vi "4Pi Astigmatism Alignment.vi"(7 "Calling VI Ref":refnum<vi>) -> ()   [LabVIEW 2016]
uses:
  Hardware Configuration/Hardware Configuration Controls/Device Type.ctl
  Hardware Configuration/Hardware Configuration Controls/Device Function.ctl
  <vilib>/Utility/miscctls.llb/LVPointTypeDef.ctl
  4Pi Astigmatism Alignment Type Defs/4Pi AA Actions.ctl
  4Pi Astigmatism Alignment Type Defs/4Pi AA Notifier Type.ctl
  Device Library/Stages/Stages Controls/Stage Actions.ctl
  <vilib>/vision/Image Controls.llb/IMAQ Image.ctl
  Device Library/Cameras/Hamamatsu/Orca Flash/Orca Flash Controls/Orca Flash Actions.ctl
  <vilib>/Analysis/NI_AALPro.lvlib
  <vilib>/Analysis/polynomials.llb/Polynomial Plot (Range).vi
  Device Library/Shutters/Shutter Controls/Shutter Actions.ctl
panel:
  in  "Scan and Align":bool
  in  "Scan Lower Obj":bool
  in  "Frame Accums.":u16=1
  in  "No. of Steps":u16=10
  in  "Step Size (µm)":dbl=0.05
  out "ROI Fit":dbl[][](graph)
  out "Image ROI":u16[][](graph)
  in  "Image Selection":i32(ring) items=["Quad 01", "Quad 02", "Quad 03", "Quad 04"]
  in  "Scan Upper Obj":bool
  in  "Quit":bool
  out "Scan Data":cluster{dbl[], dbl[]}[](graph)
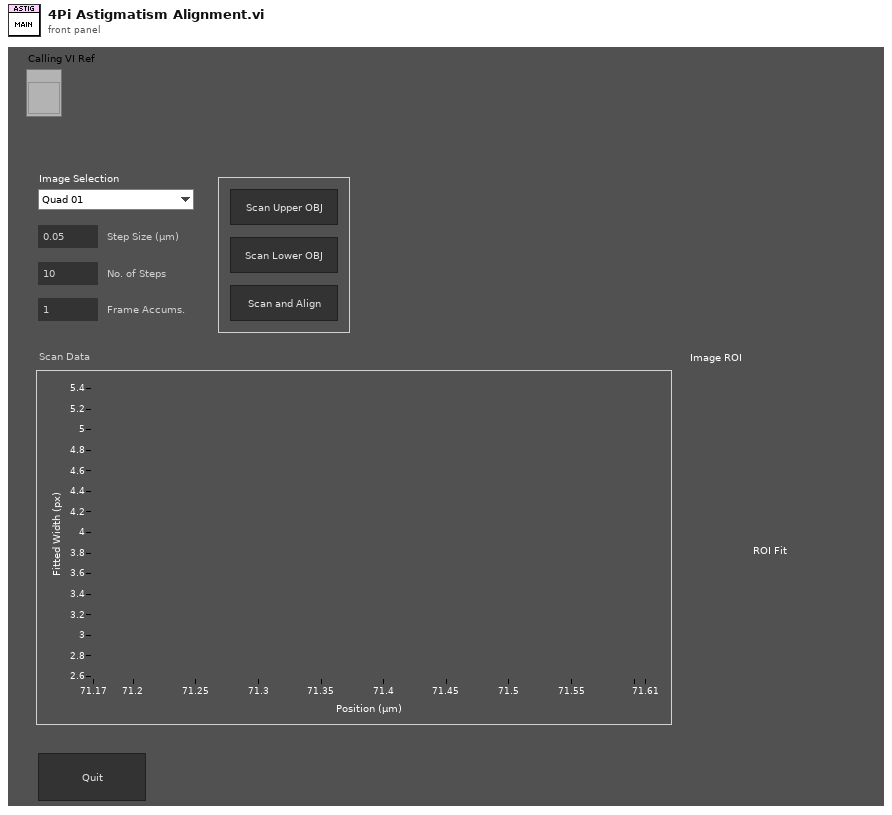
[diagram p1: front panel]
types:
  T1 = typedef "IMAQ Image.ctl" = refnum<image>
  T2 = typedef "4Pi AA Actions.ctl" = enum16{"Idle", "Scan Upper", "Scan Lower", "Scan and Align", "Open Shutter", "Close Shutter", "Set Z Start", "Get Image", "Plot Data", "Move Z Stage", "Fit Astig Curves", "Return Z Stage", "Abort", "Quit"}
  T3 = typedef "4Pi AA Notifier Type.ctl" = cluster{"Actions":T2, "Scan Steps":u16, "Step Size (µm)":dbl, "Frame Accums":u16, "Image Ref":T1, "Initial Z Pos (µm)":dbl}
  T4 = enum16{"Always On", "Always Off", "Off While Running"}
  T5 = typedef "LVPointTypeDef.ctl" = cluster{"Horizontal":i16, "Vertical":i16}
  T6 = typedef "Device Function.ctl" = enum16{"Primary", "Secondary", "Overview", "Wide Field Drift Correction", "642 nm Excitation", "560 nm Excitation", "546 nm Excitation", "488 nm Excitation", "405 nm Excitation", "Objective Drift Correction", "Objective XY", "Objective Z", "Sample XY", "Sample Coarse Z", "Sample Z", "4Pi Lower", "4Pi Upper", "Adj Cavity", "Line Scanning"}
  T7 = typedef "Device Type.ctl" = enum16{"AOTF", "Camera", "Deformable Mirror", "Laser", "Shutter", "Stage", "Waveform"}
  T8 = typedef "Orca Flash Actions.ctl" = enum16{"IDLE", "PREVIEW", "RECORD", "Record Settings", "SETPARAM", "GETPARAM", "SETROI", "GETROI", "PROGRESSIVE MODE", "AREA MODE", "STATUS", "QUIT"}
  T9 = typedef "Shutter Actions.ctl" = enum16{"Open", "Close", "Toggle", "Status", "Quit"}
  T10 = typedef "Stage Actions.ctl" = enum16{"Get Position", "MVR", "MOVE", "HALT", "ONTARGET", "ERROR", "REFERENCE", "INIT", "VELOCITY", "STATUS", "EXIT", "HOME", "ZEROPOS", "NANOPOS", "ANALOG", "QUIT"}
  T11 = enum32{"Invalid", "Standard", "Closed", "Hidden", "Minimized", "Maximized"}
  T12 = typedef "2D Gaussian - Best Fit Parameters.ctl" = cluster{"Amplitude":dbl, "X Position":dbl, "Y Position":dbl, "X Width":dbl, "Y Width":dbl, "Offset":dbl}
  T13 = typedef "LVRectTypeDef.ctl" = cluster{"Left":i16, "Top":i16, "Right":i16, "Bottom":i16}
  T14 = typedef "LVBoundsTypeDef.ctl" = cluster{"Width":u32, "Height":u32}
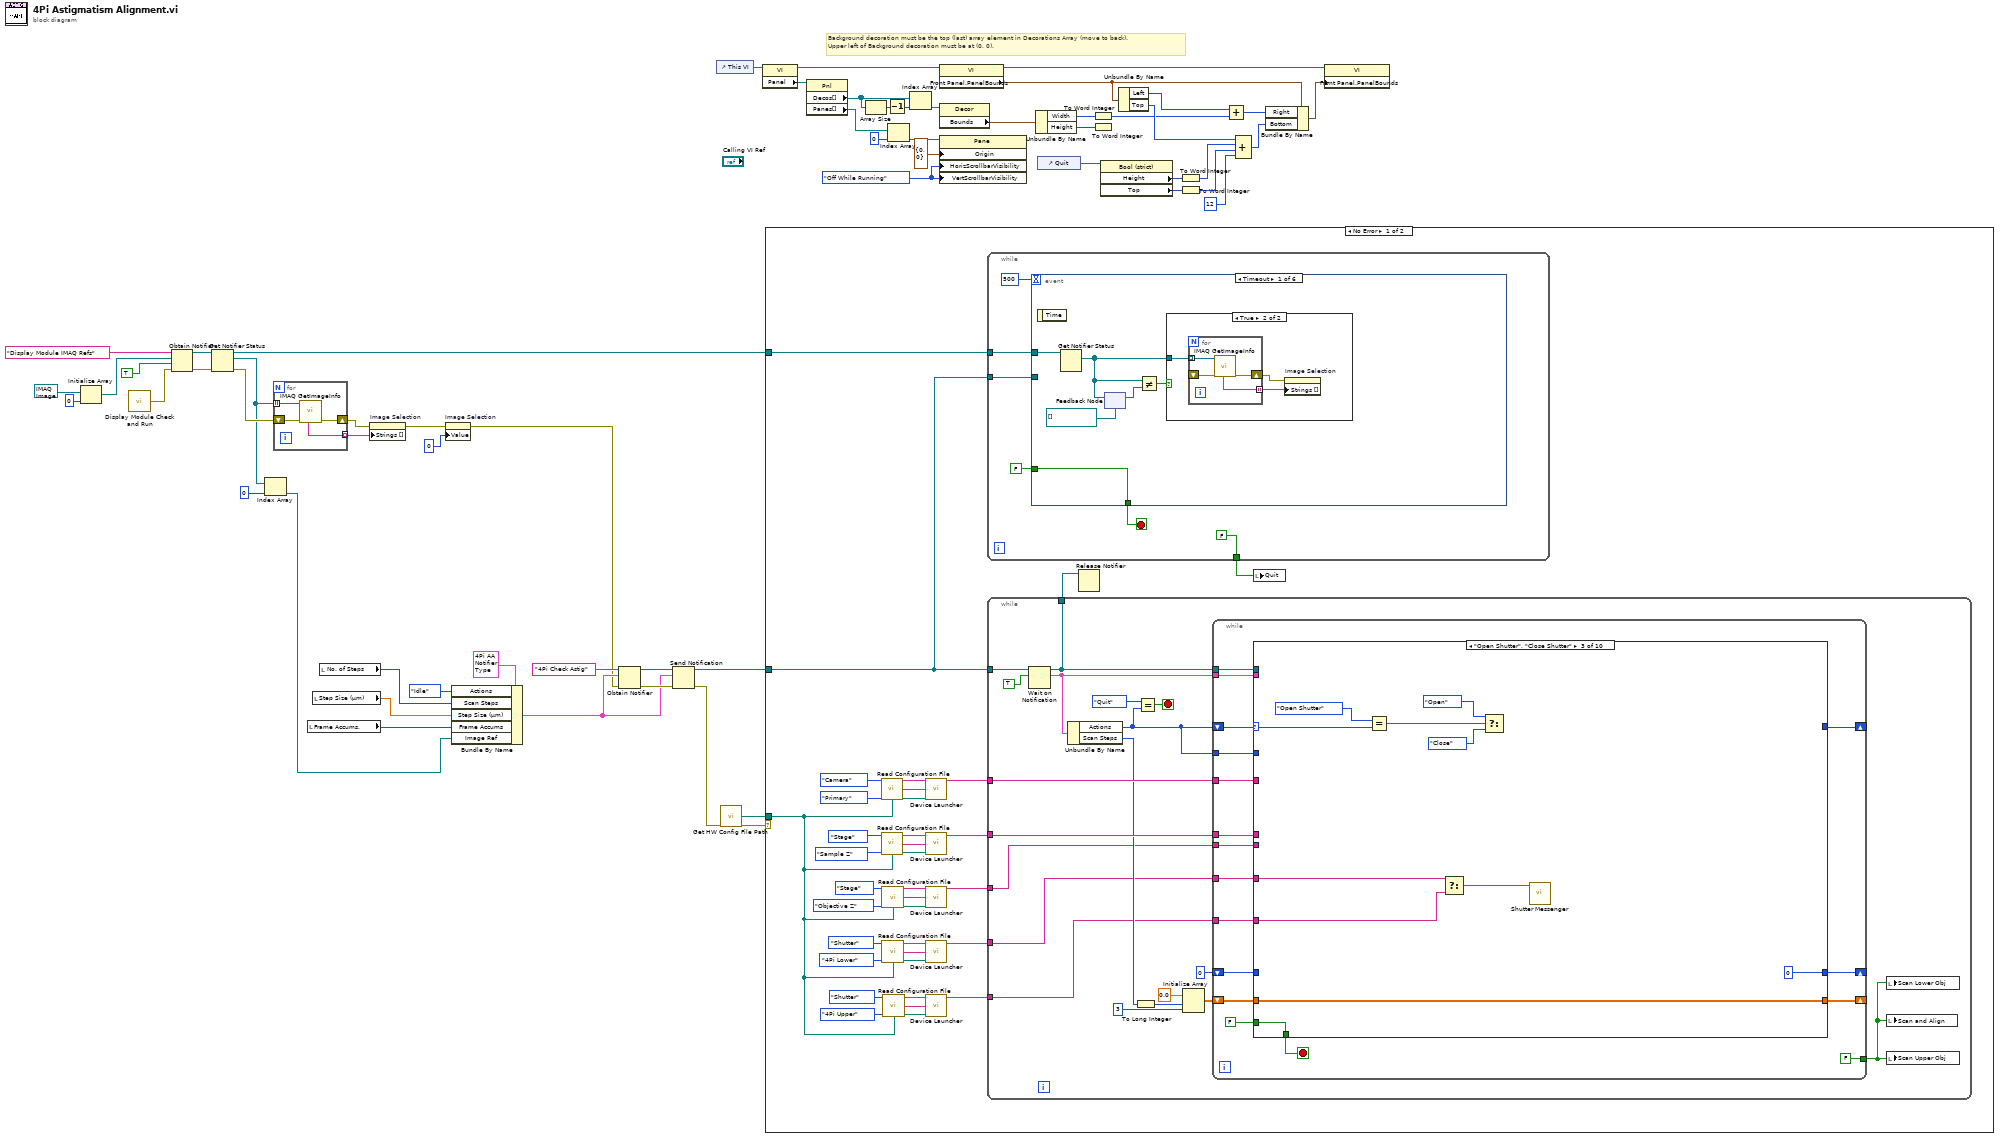
[diagram p0: block diagram]
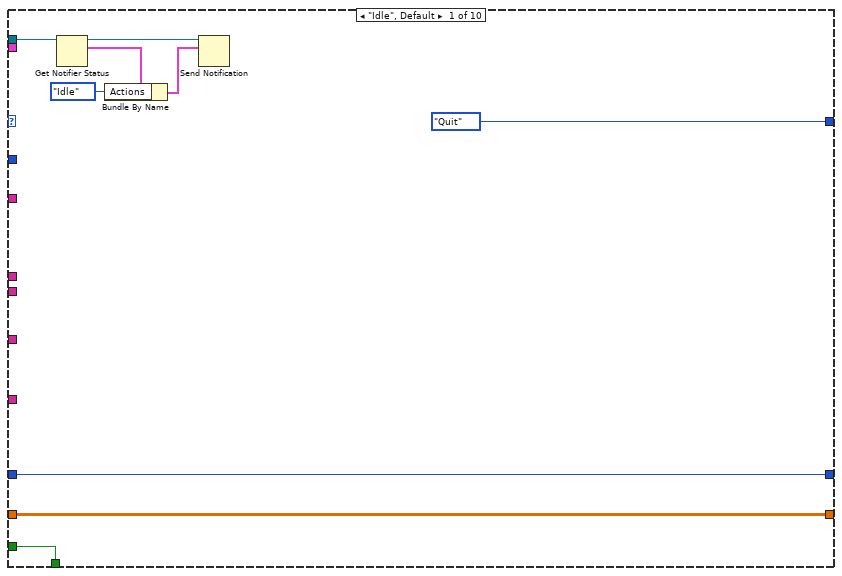
[diagram p2: hidden frame]
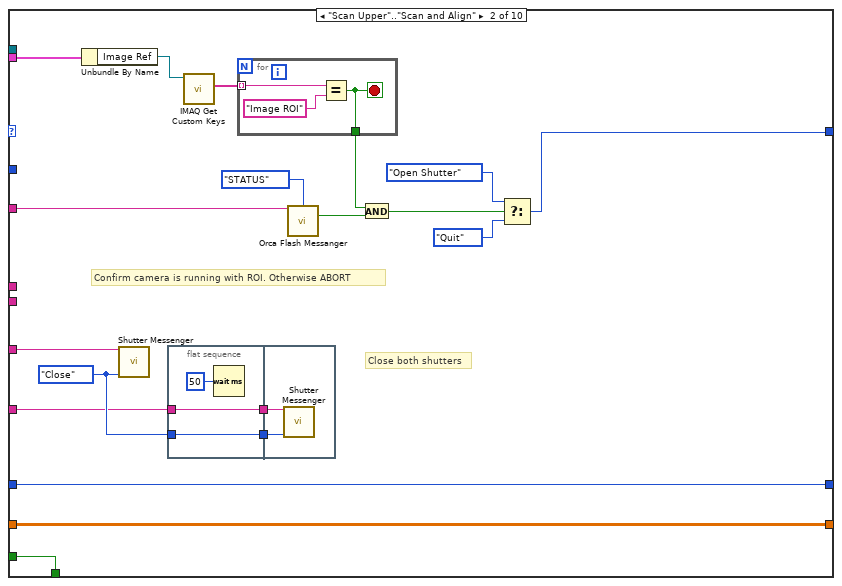
[diagram p3: hidden frame]
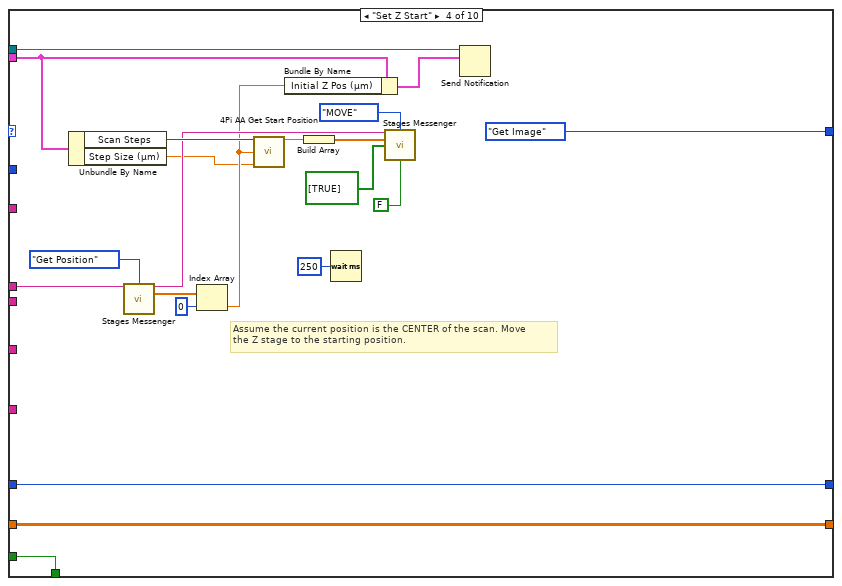
[diagram p4: hidden frame]
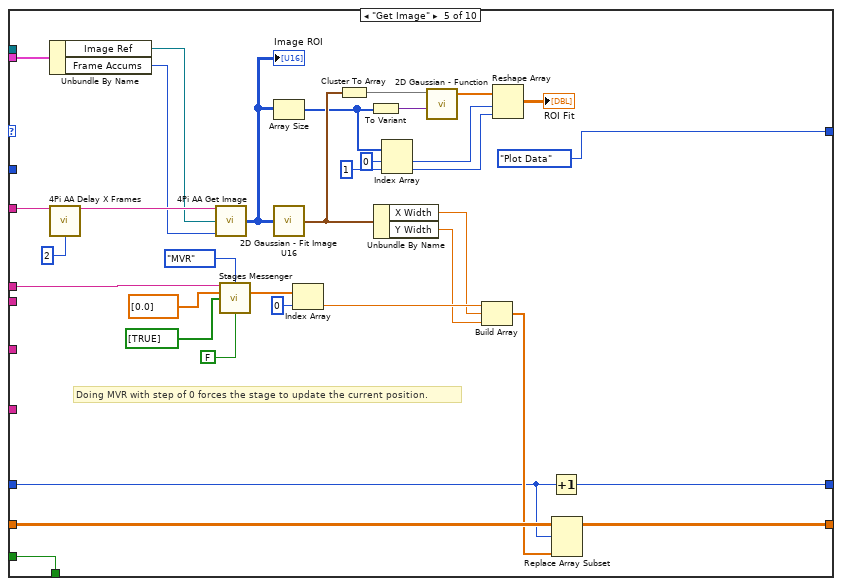
[diagram p5: hidden frame]
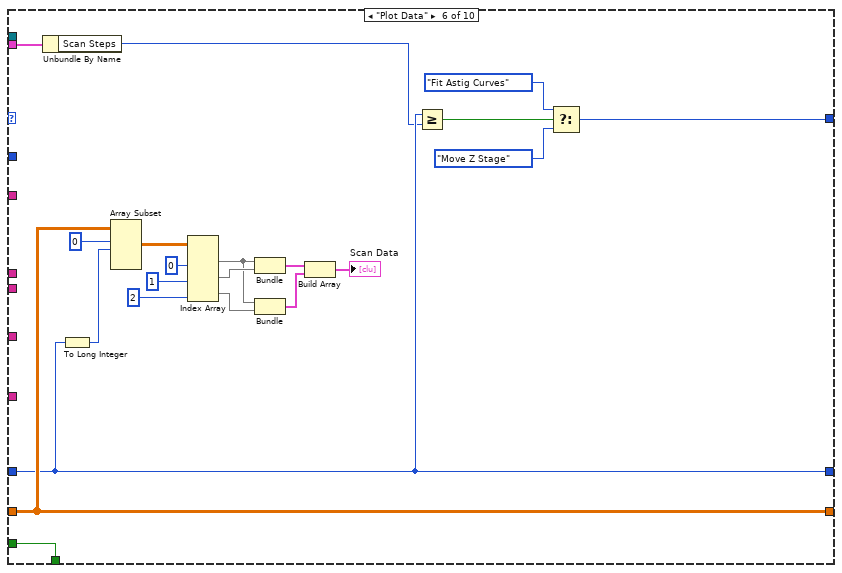
[diagram p6: hidden frame]
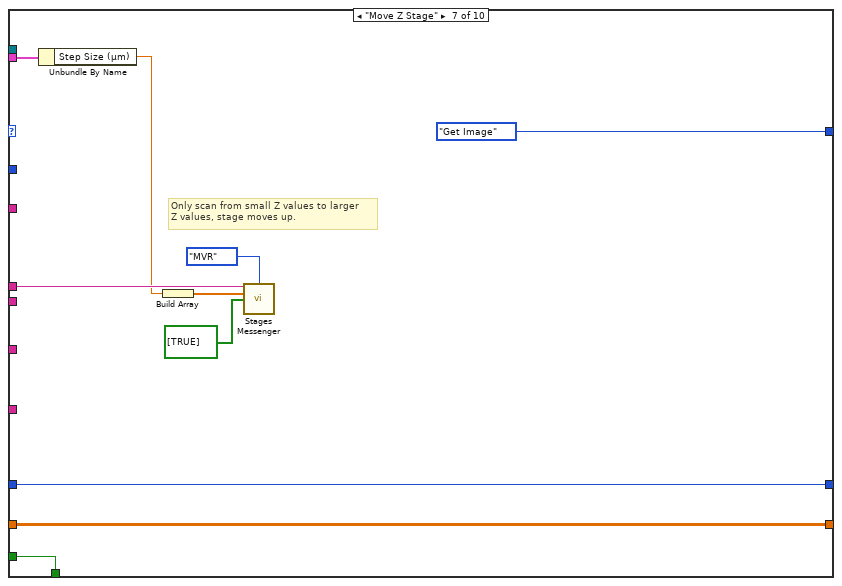
[diagram p7: hidden frame]
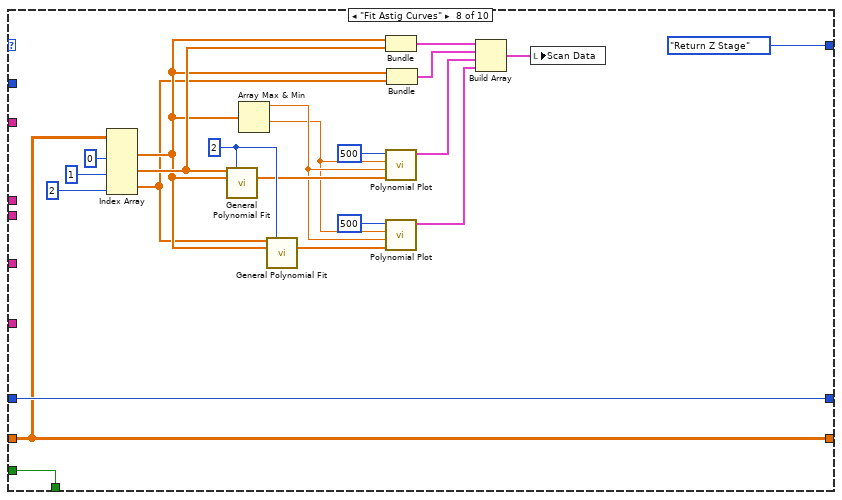
[diagram p8: hidden frame]
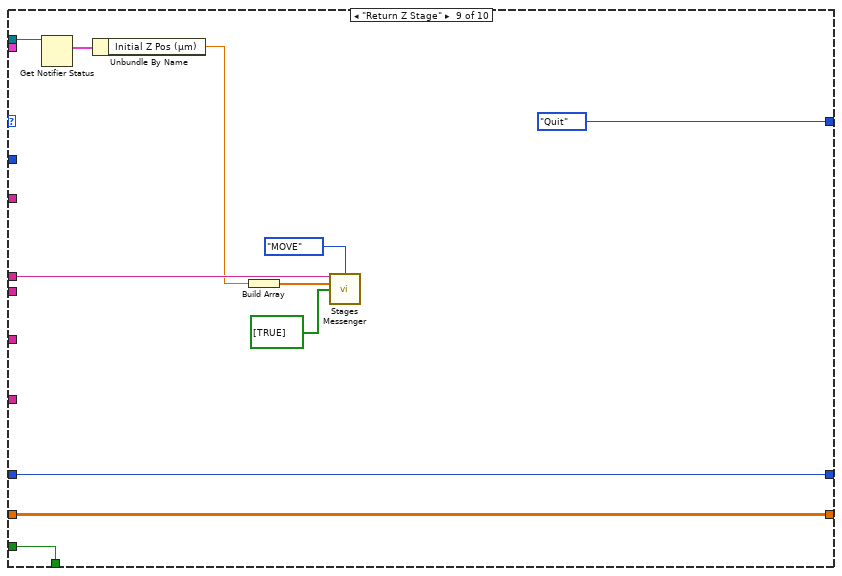
[diagram p9: hidden frame]
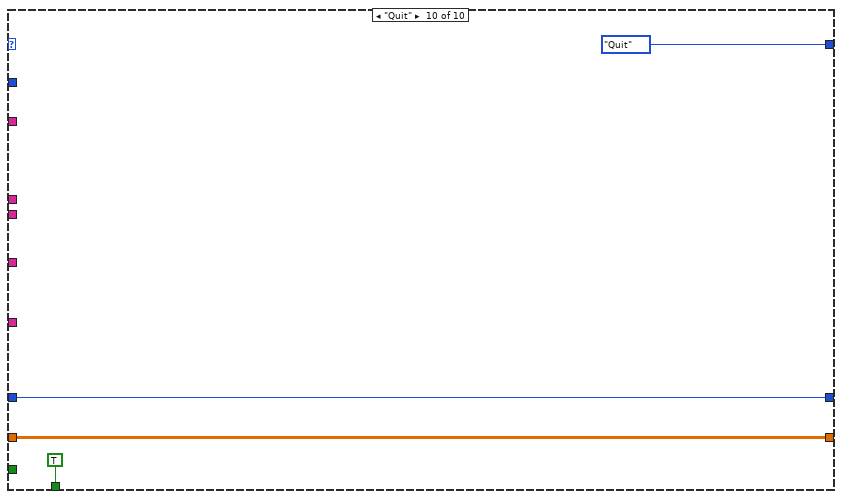
[diagram p10: hidden frame]
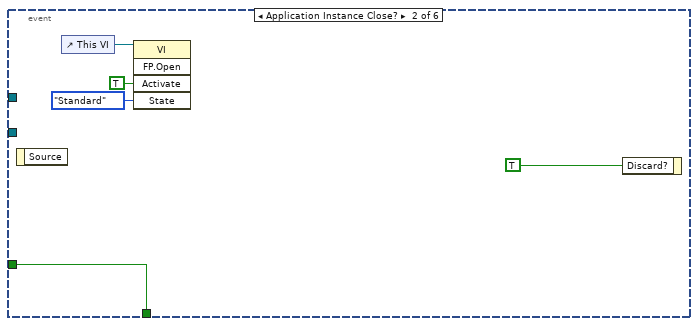
[diagram p12: hidden frame]
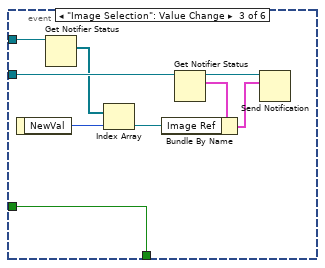
[diagram p13: hidden frame]
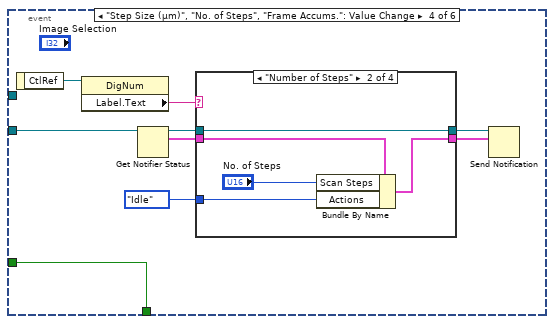
[diagram p14: hidden frame]
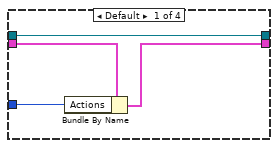
[diagram p15: hidden frame]
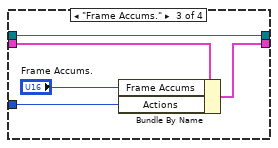
[diagram p16: hidden frame]
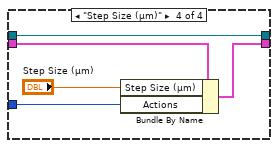
[diagram p17: hidden frame]
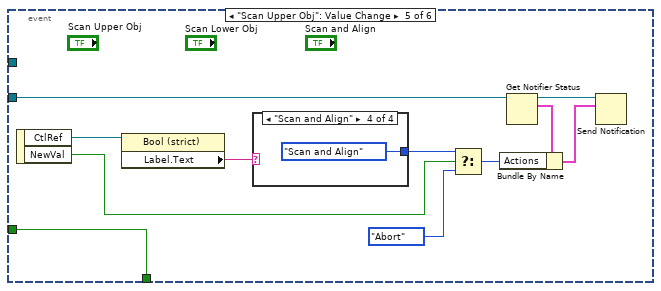
[diagram p18: hidden frame]
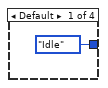
[diagram p19: hidden frame]
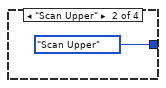
[diagram p20: hidden frame]
diagram:
  w41 = T4."Off While Running" ("Vertical Scrollbar Visibility")
  # "Background decoration must be the top (last) array element in Decorations Array (move to back).\nUpper left of Background decoration must be at (0, 0)."
  n1 = Initialize Array(T1 refnum ("New Image"), 0 ("dimension size")) -> (w17:T1[])
  n2 = call "Display Module Check and Run.vi"() -> ("Error"=w1:errorcluster)  [unwired: 15 in]
  n3 = Obtain Notifier(name (unnamed)="Display Module IMAQ Refs", notification data type=w17, create if not found? (T)=TRUE, error in (no error)=w1) -> (notifier out=w16:refnum<notifier>, error out=w15:errorcluster)  [unwired: 1 out]
  n4 = Get Notifier Status(notifier=w16, error in (no error)=w15) -> (notifier out=w14:refnum<notifier>, current notification=w8:T1[], error out=w13:errorcluster)  [unwired: 2 out]
  n5 = Index Array(array=w8, index=0) -> (element=w6:T1)
  n6 = for {
    tunnel: w8 -> [w64] mode=indexing
    shift-right: [w62] -> w11
    shift-left: w13 -> [w63]
    tunnel: [w61] -> w12 mode=indexing
    n7 = call "IMAQ GetImageInfo"("error in (no error)"=w63, "Image"=w64) -> ("error out"=w62:errorcluster, "Image Name"=w61:string)  [unwired: 2 in, 6 out]
  }
  n8 = local read "Frame Accums."() -> (w4:u16)
  n9 = local read "Step Size (µm)"() -> (w3:dbl)
  n10 = local read "No. of Steps"() -> (w2:u16)
  n11 = property on="Image Selection" class="Ring (strict)"(error in=w11, "Strings []"=w12) -> (error out=w9:errorcluster)  [unwired: 1 in, 1 out]
  n12 = property on="Image Selection" class="Ring (strict)"(error in=w9, "Value"=0) -> (error out=w5:errorcluster)  [unwired: 1 in, 1 out]
  n13 = Bundle By Name(cluster=T3 {"Actions"=enum."Idle", "Scan Steps"=1, "Step Size (µm)"=0.1, "Frame Accums"=1, "Image Ref"=refnum, "Initial Z Pos (µm)"=0.0} ("Astig Test Data Type"), "Actions"=4Pi_AA_Actions."Idle", "Scan Steps"=w2, "Step Size (µm)"=w3, "Frame Accums"=w4, "Image Ref"=w6) -> (w22:T3)
  n14 = Obtain Notifier(name (unnamed)="4Pi Check Astig", notification data type=w22, error in (no error)=w5) -> (notifier out=w29:refnum<notifier>, error out=w28:errorcluster)  [unwired: 1 in, 1 out]
  n15 = Send Notification(notification=w22, notifier=w29, error in (no error)=w28) -> (notifier out=w25:refnum<notifier>, error out=w26:errorcluster)
  n16 = control-ref of="This VI"() -> (w33:refnum<vi>)
  n17 = call "Get HW Config File Path.vi"("Error"=w26) -> ("File Path"=w59:path, "Error"=w60:errorcluster)  [unwired: 13 in]
  n18 = property class="VI"(reference=w33) -> (reference out=w42:refnum<vi>, "Panel"=w34:refnum<vi>)  [unwired: 1 in, 1 out]
  n19 = case shown="No Error" w60 {
    tunnel: w59 -> [w66 _]
    tunnel: w25 -> [w87 _]
    tunnel: w14 -> [w84 _]
    frame No Error {
      n20 = call "Read Configuration File.vi"("Device Type"=Device_Type."Camera", "Device Function"=Device_Function."Primary", "Config File Path"=w66) -> ("Unique Notifier Name"=w97:string, "Device Ports/IDs/Channels"=w99:string[], "Device Engine Path"=w98:path)  [unwired: 9 in, 1 out]
      n21 = call "Read Configuration File.vi"("Device Type"=Device_Type."Stage", "Device Function"=Device_Function."Sample Z", "Config File Path"=w66) -> ("Unique Notifier Name"=w91:string, "Device Ports/IDs/Channels"=w89:string[], "Device Engine Path"=w90:path)  [unwired: 9 in, 1 out]
      n22 = call "Read Configuration File.vi"("Device Type"=Device_Type."Stage", "Device Function"=Device_Function."Objective Z", "Config File Path"=w66) -> ("Unique Notifier Name"=w74:string, "Device Ports/IDs/Channels"=w75:string[], "Device Engine Path"=w76:path)  [unwired: 9 in, 1 out]
      n23 = call "Read Configuration File.vi"("Device Type"=Device_Type."Shutter", "Device Function"=Device_Function."4Pi Lower", "Config File Path"=w66) -> ("Unique Notifier Name"=w83:string, "Device Ports/IDs/Channels"=w82:string[], "Device Engine Path"=w81:path)  [unwired: 9 in, 1 out]
      n24 = call "Read Configuration File.vi"("Device Type"=Device_Type."Shutter", "Device Function"=Device_Function."4Pi Upper", "Config File Path"=w66) -> ("Unique Notifier Name"=w67:string, "Device Ports/IDs/Channels"=w68:string[], "Device Engine Path"=w69:path)  [unwired: 9 in, 1 out]
      n25 = call "Device Launcher.vi"("Notifier Name"=w97, "Device Ports/IDs/Channels"=w99, "Device Engine Path"=w98) -> ("Notifier Name"=w85:string)  [unwired: 11 in, 1 out]
      n26 = call "Device Launcher.vi"("Notifier Name"=w91, "Device Ports/IDs/Channels"=w89, "Device Engine Path"=w90) -> ("Notifier Name"=w86:string)  [unwired: 11 in, 1 out]
      n27 = call "Device Launcher.vi"("Notifier Name"=w74, "Device Ports/IDs/Channels"=w75, "Device Engine Path"=w76) -> ("Notifier Name"=w73:string)  [unwired: 11 in, 1 out]
      n28 = call "Device Launcher.vi"("Notifier Name"=w83, "Device Ports/IDs/Channels"=w82, "Device Engine Path"=w81) -> ("Notifier Name"=w72:string)  [unwired: 11 in, 1 out]
      n29 = call "Device Launcher.vi"("Notifier Name"=w67, "Device Ports/IDs/Channels"=w68, "Device Engine Path"=w69) -> ("Notifier Name"=w65:string)  [unwired: 11 in, 1 out]
      n30 = while {
        tunnel: [FALSE] -> w94
        tunnel: w87 -> [w307]
        tunnel: w84 -> [w306]
        stop <- w309 stop-if-true
        n31 = event shown="[0] Timeout" {
          selector: _ -> [_ _ _ _ _ _]
          dyn-events: _ -> [_ _ _ _ _ _]
          timeout: 500 -> [_ _ _ _ _ _]
          tunnel: FALSE -> [w317 w328 w338 w347 w377 _]
          tunnel: [w317 w328 w338 w347 w377 w387] -> w309
          tunnel: w307 -> [_ _ w337 w346 w376 w382]
          tunnel: w306 -> [w316 _ w333 _ _ _]
          event Timeout {
            n32 = event-data() -> ()  [unwired: 1 in, 1 out]
            n33 = Get Notifier Status(notifier=w316) -> (current notification=w312:T1[])  [unwired: 1 in, 4 out]
            n34 = feedback-in #1(w312) -> ()
            n35 = feedback #1(T1[] []) -> (w314:T1[])
            n36 = Not Equal?(x=w312, y=w314) -> (x != y?=w313:bool)
            n37 = case shown="True" w313 {
              tunnel: w312 -> [_ w318]
              frame False {
              }
              frame True {
                n38 = for {
                  tunnel: w318 -> [w324] mode=indexing
                  shift-right: [w322] -> w319
                  shift-left: _ -> [w323]
                  tunnel: [w321] -> w320 mode=indexing
                  n39 = call "IMAQ GetImageInfo"("error in (no error)"=w323, "Image"=w324) -> ("error out"=w322:errorcluster, "Image Name"=w321:string)  [unwired: 2 in, 6 out]
                }
                n40 = property on="Image Selection" class="Ring (strict)"(error in=w319, "Strings []"=w320) -> ()  [unwired: 1 in, 2 out]
              }
            }
          }
          event Application Instance Close? {
            n41 = event-data() -> ()  [unwired: 1 in, 1 out]
            n42 = control-ref of="This VI"() -> (w325:refnum<vi>)
            n43 = invoke class="VI" method="FP.Open"(reference=w325, "Activate"=TRUE ("Activate?"), "State"=T11."Standard") -> ()  [unwired: 2 in, 5 out]
            n44 = event-data("Discard?"=TRUE) -> ()  [unwired: 1 in, 1 out]
          }
          event "Image Selection": Value Change {
            n45 = event-data() -> ("NewVal"=w330:i32)  [unwired: 1 in]
            n46 = Get Notifier Status(notifier=w333) -> (current notification=w332:T1[])  [unwired: 1 in, 4 out]
            n47 = Index Array(array=w332, index=w330) -> (element=w331:T1)
            n48 = Get Notifier Status(notifier=w337) -> (notifier out=w336:refnum<notifier>, current notification=w335:T3)  [unwired: 1 in, 3 out]
            n49 = Bundle By Name(cluster=w335, "Image Ref"=w331) -> (w334:T3)
            n50 = Send Notification(notification=w334, notifier=w336) -> ()  [unwired: 1 in, 2 out]
          }
          event "Step Size (µm)", "No. of Steps", "Frame Accums.": Value Change {
            n51 = event-data() -> ("CtlRef"=w345:refnum<vi>)  [unwired: 1 in]
            n52 = property class="DigNum"(reference=w345) -> ("Label.Text"=w344:string)  [unwired: 1 in, 2 out]
            n53 = Get Notifier Status(notifier=w346) -> (notifier out=w343:refnum<notifier>, current notification=w342:T3)  [unwired: 1 in, 3 out]
            n54 = case shown="\"Number of Steps\"" w344 {
              tunnel: w343 -> [w351 w356 w361 w366]
              tunnel: w342 -> [w350 w355 w360 w365]
              tunnel: [w351 w356 w361 w366] -> w341
              tunnel: [w349 w354 w359 w364] -> w340
              tunnel: 4Pi_AA_Actions."Idle" ("Actions") -> [w348 w353 w358 w363]
              frame Default {
                n55 = Bundle By Name(cluster=w350, "Actions"=w348) -> (w349:T3)
              }
              frame "Number of Steps" {
                n56 = Bundle By Name(cluster=w355, "Scan Steps"="No. of Steps", "Actions"=w353) -> (w354:T3)
              }
              frame "Frame Accums." {
                n57 = Bundle By Name(cluster=w360, "Frame Accums"="Frame Accums.", "Actions"=w358) -> (w359:T3)
              }
              frame "Step Size (µm)" {
                n58 = Bundle By Name(cluster=w365, "Step Size (µm)"="Step Size (µm)", "Actions"=w363) -> (w364:T3)
              }
            }
            n59 = Send Notification(notification=w340, notifier=w341) -> ()  [unwired: 1 in, 2 out]
          }
          event "Scan Upper Obj": Value Change {
            n60 = event-data() -> ("CtlRef"=w372:refnum<vi>, "NewVal"=w368:bool)  [unwired: 1 in]
            n61 = property class="Bool (strict)"(reference=w372) -> ("Label.Text"=w371:string)  [unwired: 1 in, 2 out]
            n62 = case shown="\"Scan and Align\"" w371 {
              tunnel: [4Pi_AA_Actions."Idle" ("Actions") 4Pi_AA_Actions."Scan Upper" ("Actions") 4Pi_AA_Actions."Scan Lower" ("Actions") 4Pi_AA_Actions."Scan and Align" ("Actions")] -> w370
              frame Default {
              }
              frame "Scan Upper" {
              }
              frame "Scan Lower" {
              }
              frame "Scan and Align" {
              }
            }
            n63 = Select(t=w370, s=w368, f=4Pi_AA_Actions."Abort" ("Actions")) -> (s? t:f=w369:T2)
            n64 = Get Notifier Status(notifier=w376) -> (notifier out=w375:refnum<notifier>, current notification=w374:T3)  [unwired: 1 in, 3 out]
            n65 = Bundle By Name(cluster=w374, "Actions"=w369) -> (w373:T3)
            n66 = Send Notification(notification=w373, notifier=w375) -> ()  [unwired: 1 in, 2 out]
          }
          event "Quit": Value Change {
            n67 = event-data() -> ("NewVal"=w387:bool)  [unwired: 1 in]
            n68 = Get Notifier Status(notifier=w382) -> (notifier out=w386:refnum<notifier>, current notification=w385:T3)  [unwired: 1 in, 3 out]
            n69 = Bundle By Name(cluster=w385, "Actions"=4Pi_AA_Actions."Quit") -> (w384:T3)
            n70 = Send Notification(notification=w384, notifier=w386) -> ()  [unwired: 1 in, 2 out]
          }
        }
      }
      n71 = while {
        tunnel: w87 -> [w118]
        tunnel: [w114] -> w88
        tunnel: w86 -> [w113]
        tunnel: w85 -> [w111]
        tunnel: w73 -> [w102]
        tunnel: w72 -> [w101]
        tunnel: w65 -> [w100]
        stop <- w116 stop-if-true
        n72 = Wait on Notification(notifier=w118, ignore previous (F)=TRUE) -> (notifier out=w114:refnum<notifier>, notification=w115:T3)  [unwired: 2 in, 2 out]
        n73 = Unbundle By Name(w115) -> ("Actions"=w103:T2, "Scan Steps"=w109:u16)
        n74 = To Long Integer(number=w109) -> (32bit integer=w106:i32)
        n75 = Equal?(x=4Pi_AA_Actions."Quit" ("y"), y=w103) -> (x = y?=w116:bool)
        n76 = Initialize Array(0.0 ("element"), w106, 3 ("dimension size")) -> (w107:dbl[][])
        n77 = while {
          tunnel: w115 -> [w132]
          shift-right: [w129] -> _
          shift-left: w103 -> [w135]
          tunnel: w114 -> [w131]
          tunnel: w113 -> [w130]
          shift-right: [w127] -> _
          shift-left: u16 0 -> [w128]
          tunnel: w111 -> [w126]
          shift-right: [w124] -> _
          shift-left: w107 -> [w125]
          tunnel: [FALSE] -> w104
          tunnel: w103 -> [w122]
          tunnel: w102 -> [w121]
          tunnel: w101 -> [w120]
          tunnel: w100 -> [w119]
          stop <- w133 stop-if-true
          n78 = case shown="\"Open Shutter\", \"Close Shutter\"" w135 {
            selector: w135 -> [_ _ w179 _ _ _ _ _ _ _]
            tunnel: FALSE -> [w144 w163 w182 w198 w237 w258 w268 w290 w298 _]
            tunnel: [w144 w163 w182 w198 w237 w258 w268 w290 w298 TRUE] -> w133
            tunnel: w132 -> [_ w160 _ w192 w233 w255 w261 _ _ _]
            tunnel: w131 -> [w143 _ _ w193 _ _ _ _ w294 _]
            tunnel: w130 -> [_ _ _ w202 w228 _ w263 _ w295 _]
            tunnel: [4Pi_AA_Actions."Quit" ("y") w152 _ 4Pi_AA_Actions."Get Image" ("y") 4Pi_AA_Actions."Plot Data" ("y") w250 4Pi_AA_Actions."Get Image" ("y") 4Pi_AA_Actions."Return Z Stage" ("y") 4Pi_AA_Actions."Quit" ("y") 4Pi_AA_Actions."Quit" ("y")] -> w129
            tunnel: [w136 w151 u16 0 w195 w219 w254 w267 w289 w300 w304] -> w127
            tunnel: w128 -> [w136 w151 _ w195 w218 w254 w267 w289 w300 w304]
            tunnel: w126 -> [_ w162 _ _ w236 _ _ _ _ _]
            tunnel: w125 -> [w137 w150 w181 w194 w223 w257 w259 w287 w299 w303]
            tunnel: [w137 w150 w181 w194 w222 w257 w259 w287 w299 w303] -> w124
            tunnel: w122 -> [_ _ _ _ _ _ _ _ _ _]
            tunnel: w121 -> [_ _ _ _ _ _ _ _ _ _]
            tunnel: w120 -> [_ w145 w174 _ _ _ _ _ _ _]
            tunnel: w119 -> [_ w146 w173 _ _ _ _ _ _ _]
            frame "Idle", Default {
              n79 = Get Notifier Status(notifier=w143) -> (notifier out=w142:refnum<notifier>, current notification=w141:T3)  [unwired: 1 in, 3 out]
              n80 = Bundle By Name(cluster=w141, "Actions"=4Pi_AA_Actions."Idle") -> (w139:T3)
              n81 = Send Notification(notification=w139, notifier=w142) -> ()  [unwired: 1 in, 2 out]
            }
            frame "Scan Upper".."Scan and Align" {
              w147 = Shutter_Actions."Close" ("Action")
              # "Close both shutters"
              # "Confirm camera is running with ROI. Otherwise ABORT"
              n82 = Unbundle By Name(w160) -> ("Image Ref"=w158:T1)
              n83 = call "Shutter Messenger.vi"("Notifier Name"=w145, "Action"=w147) -> ()  [unwired: 12 in, 2 out]
              n84 = flat-sequence {
                tunnel: w147 -> [w165]
                tunnel: w146 -> [w166]
                tunnel: [w166] -> w149
                tunnel: [w165] -> w148
                tunnel: w149 -> [w168]
                tunnel: w148 -> [w167]
                frame #0 {
                  n85 = Wait (ms)(milliseconds to wait=u32 50) -> ()  [unwired: 1 out]
                }
                frame #1 {
                  n86 = call "Shutter Messenger.vi"("Notifier Name"=w168, "Action"=w167) -> ()  [unwired: 12 in, 2 out]
                }
              }
              n87 = call "IMAQ Get Custom Keys"("Image"=w158) -> ("Keys"=w159:string[])  [unwired: 7 in, 3 out]
              n88 = for {
                tunnel: w159 -> [w171] mode=indexing
                tunnel: [w169] -> w156
                stop <- w169 stop-if-true
                n89 = Equal?(x=w171, y="Image ROI") -> (x = y?=w169:bool)
              }
              n90 = call "Orca Flash Messanger.vi"("Notifier Name"=w162, "Camera Actions"=Orca_Flash_Actions."STATUS") -> ("Running?"=w157:bool)  [unwired: 9 in, 4 out]
              n91 = And(x=w156, y=w157) -> (x .and. y?=w155:bool)
              n92 = Select(t=4Pi_AA_Actions."Open Shutter" ("y"), s=w155, f=4Pi_AA_Actions."Quit") -> (s? t:f=w152:T2)
            }
            frame "Open Shutter", "Close Shutter" {
              n93 = Equal?(x=4Pi_AA_Actions."Open Shutter", y=w179) -> (x = y?=w177:bool)
              n94 = Select(t=w174, f=w173) -> (s? t:f=w172:string)  [unwired: 1 in]
              n95 = Select(t=Shutter_Actions."Open" ("Action"), s=w177, f=Shutter_Actions."Close" ("Action")) -> ()  [unwired: 1 out]
              n96 = call "Shutter Messenger.vi"("Notifier Name"=w172) -> ()  [unwired: 13 in, 2 out]
            }
            frame "Set Z Start" {
              # "Assume the current position is the CENTER of the scan. Move\nthe Z stage to the starting position."
              n97 = Unbundle By Name(w192) -> ("Scan Steps"=w203:u16, "Step Size (µm)"=w184:dbl)
              n98 = call "Stages Messenger.vi"("Stage Notifier Name"=w202, "Actions"=Stage_Actions."Get Position") -> ("Stage Notifier Name (Dup)"=w197:string, "Positions"=w200:dbl[])  [unwired: 10 in, 2 out]
              n99 = Index Array(array=w200, index=0) -> (element=w190:dbl)
              n100 = call "4Pi AA Get Start Position.vi"("Number of Steps"=w203, "Center Value"=w190, "Step Size"=w184) -> ("Starting Value"=w189:dbl)  [unwired: 11 in, 1 out]
              n101 = Bundle By Name(cluster=w192, "Initial Z Pos (µm)"=w190) -> (w191:T3)
              n102 = Build Array(w189) -> (w187:dbl[])
              n103 = Wait (ms)(milliseconds to wait=u32 250) -> ()  [unwired: 1 out]
              n104 = call "Stages Messenger.vi"("Stage Notifier Name"=w197, "Actions"=Stage_Actions."MOVE", "Setpoint"=w187, "Axis"=bool[] [TRUE], "Exit While Busy?"=FALSE) -> ()  [unwired: 7 in, 4 out]
              n105 = Send Notification(notification=w191, notifier=w193) -> ()  [unwired: 1 in, 2 out]
            }
            frame "Get Image" {
              # "Doing MVR with step of 0 forces the stage to update the current position."
              n106 = Unbundle By Name(w233) -> ("Image Ref"=w224:T1, "Frame Accums"=w232:u16)
              n107 = call "4Pi AA Delay X Frames.vi"("Camera Notifier Name"=w236, "Wait No. (1)"=u32 2) -> ("Camera Notifier Name (Dup)"=w234:string)  [unwired: 13 in]
              n108 = call "4Pi AA Get Image.vi"("Camera Notifier Name"=w234, "Image Ref"=w224, "Frame Accums."=w232) -> ("Image Out"=w214:u16[][])  [unwired: 12 in]
              "Image ROI" <- w214
              n109 = call "Stages Messenger.vi"("Stage Notifier Name"=w228, "Actions"=Stage_Actions."MVR", "Setpoint"=dbl[] [0.0], "Axis"=bool[] [TRUE], "Exit While Busy?"=FALSE) -> ("Positions"=w230:dbl[])  [unwired: 7 in, 3 out]
              n110 = Array Size(array=w214) -> (size(s)=w209:i32[])
              n111 = call "2D Gaussian - Fit Image U16.vi"("Image In (U16)"=w214) -> ("Best Fit Params"=w212:T12)  [unwired: 14 in]
              n112 = Index Array(array=w230, index=0) -> (element=w227:dbl)
              n113 = Cluster To Array(cluster=w212) -> (array=w211:dbl[])
              n114 = To Variant(anything=w209) -> (Variant=w213:variant)
              n115 = Unbundle By Name(w212) -> ("X Width"=w225:dbl, "Y Width"=w226:dbl)
              n116 = Index Array(array=w209, index #1=0 ("index"), index #2=1 ("index")) -> (element #1=w206:i32, element #2=w205:i32)
              n117 = call "2D Gaussian - Function.vi"("data"=w213, "a"=w211) -> ("f(X,a)"=w210:dbl[])  [unwired: 2 in, 2 out]
              n118 = Build Array(w227, w225, w226) -> (w221:dbl[])
              n119 = Reshape Array(w210, w206, w205) -> (→"ROI Fit":dbl[][])
              n120 = Increment(x=w218) -> (x+1=w219:u16)
              n121 = Replace Array Subset(array=w223, new element=w221, index (row)=w218) -> (w222:dbl[][])  [unwired: 1 in]
            }
            frame "Plot Data" {
              n122 = Unbundle By Name(w255) -> ("Scan Steps"=w253:u16)
              n123 = To Long Integer(number=w254) -> (32bit integer=w238:i32)
              n124 = Array Subset(array=w257, index (row)=0 ("index"), length (row)=w238) -> (w248:dbl[][])  [unwired: 2 in]
              n125 = Index Array(array=w248, index (col) #1=0 ("disabled index (col)"), index (col) #2=1 ("index (col)"), index (col) #3=2 ("index (col)")) -> (element #1=w242:dbl[], element #2=w244:dbl[], element #3=w243:dbl[])  [unwired: 3 in]
              n126 = Bundle(w242, w244) -> (w241:cluster{dbl[], dbl[]})  [unwired: 1 in]
              n127 = Bundle(w242, w243) -> (w240:cluster{dbl[], dbl[]})  [unwired: 1 in]
              n128 = Build Array(w241, w240) -> (→"Scan Data":cluster{dbl[], dbl[]}[])
              n129 = Greater Or Equal?(x=w254, y=w253) -> (x >= y?=w252:bool)
              n130 = Select(t=4Pi_AA_Actions."Fit Astig Curves" ("y"), s=w252, f=4Pi_AA_Actions."Move Z Stage" ("y")) -> (s? t:f=w250:T2)
            }
            frame "Move Z Stage" {
              # "Only scan from small Z values to larger\nZ values, stage moves up."
              n131 = Unbundle By Name(w261) -> ("Step Size (µm)"=w260:dbl)
              n132 = Build Array(w260) -> (w265:dbl[])
              n133 = call "Stages Messenger.vi"("Stage Notifier Name"=w263, "Actions"=Stage_Actions."MVR", "Setpoint"=w265, "Axis"=bool[] [TRUE]) -> ()  [unwired: 8 in, 4 out]
            }
            frame "Fit Astig Curves" {
              w283 = 2 ("polynomial order")
              n134 = Index Array(array=w287, index (col) #1=0 ("disabled index (col)"), index (col) #2=1 ("index (col)"), index (col) #3=2 ("index (col)")) -> (element #1=w275:dbl[], element #2=w276:dbl[], element #3=w274:dbl[])  [unwired: 3 in]
              n135 = call <vilib>:"General Polynomial Fit.vi"("Y"=w276, "polynomial order"=w283, "X"=w275) -> ("Polynomial Coefficients"=w282:dbl[])  [unwired: 9 in, 3 out]
              n136 = Array Max & Min(array=w275) -> (max value=w278:dbl, min value=w277:dbl)  [unwired: 2 out]
              n137 = call <vilib>:"General Polynomial Fit.vi"("Y"=w274, "polynomial order"=w283, "X"=w275) -> ("Polynomial Coefficients"=w279:dbl[])  [unwired: 9 in, 3 out]
              n138 = Bundle(w275, w276) -> (w273:cluster{dbl[], dbl[]})  [unwired: 1 in]
              n139 = call-poly <vilib>:"Polynomial Plot.vi"("P(x)"=w282, "end"=w278, "start"=w277, "samples"=500) -> ("polynomial plot"=w271:cluster{"Ramp Pattern":dbl[], "P(A)":dbl[]})  [unwired: 6 in, 1 out]
              n140 = call-poly <vilib>:"Polynomial Plot.vi"("P(x)"=w279, "end"=w278, "start"=w277, "samples"=500) -> ("polynomial plot"=w270:cluster{"Ramp Pattern":dbl[], "P(A)":dbl[]})  [unwired: 6 in, 1 out]
              n141 = Bundle(w275, w274) -> (w272:cluster{dbl[], dbl[]})  [unwired: 1 in]
              n142 = Build Array(w273, w272, w271, w270) -> (w269:cluster{"Ramp Pattern":dbl[], "P(A)":dbl[]}[])
              n143 = local write "Scan Data"(w269) -> ()
            }
            frame "Return Z Stage" {
              n144 = Get Notifier Status(notifier=w294) -> (current notification=w293:T3)  [unwired: 1 in, 4 out]
              n145 = Unbundle By Name(w293) -> ("Initial Z Pos (µm)"=w292:dbl)
              n146 = Build Array(w292) -> (w291:dbl[])
              n147 = call "Stages Messenger.vi"("Stage Notifier Name"=w295, "Actions"=Stage_Actions."MOVE", "Setpoint"=w291, "Axis"=bool[] [TRUE]) -> ()  [unwired: 8 in, 4 out]
            }
            frame "Quit" {
            }
          }
        }
        n148 = local write "Scan Lower Obj"(w104) -> ()
        n149 = local write "Scan and Align"(w104) -> ()
        n150 = local write "Scan Upper Obj"(w104) -> ()
      }
      n151 = Release Notifier(notifier=w88) -> ()  [unwired: 2 in, 3 out]
      n152 = local write "Quit"(w94) -> ()
    }
    frame Error {
    }
  }
  n153 = property class="Pnl"(reference=w34) -> ("Decos[]"=w32:refnum<vi>[], "Panes[]"=w38:refnum<vi>[])  [unwired: 1 in, 2 out]
  n154 = Array Size(array=w32) -> (size(s)=w30:i32)
  n155 = Decrement(x=w30) -> (x-1=w31:i32)
  n156 = Index Array(array=w38, index=0) -> (element=w37:refnum<vi>)
  n157 = Index Array(array=w32, index=w31) -> (element=w40:refnum<vi>)
  n158 = property class="VI"(reference=w42) -> (reference out=w44:refnum<vi>, "Front Panel.PanelBounds"=w45:T13)  [unwired: 1 in, 1 out]
  n159 = property class="Decor"(reference=w40) -> ("Bounds"=w43:T14)  [unwired: 1 in, 2 out]
  n160 = property class="Pane"(reference=w37, "Origin"=T5 {"Horizontal"=0, "Vertical"=0}, "HorizScrollbarVisibility"=w41, "VertScrollbarVisibility"=w41) -> ()  [unwired: 1 in, 2 out]
  n161 = Unbundle By Name(w43) -> ("Width"=w48:u32, "Height"=w51:u32)
  n162 = control-ref of="Quit"() -> (w35:refnum<vi>)
  n163 = To Word Integer(number=w48) -> (16bit integer=w50:i16)
  n164 = To Word Integer(number=w51) -> ()  [unwired: 1 out]
  n165 = property class="Bool (strict)"(reference=w35) -> ("Height"=w53:u32, "Top"=w54:i32)  [unwired: 1 in, 2 out]
  n166 = Unbundle By Name(w45) -> ("Left"=w47:i16, "Top"=w58:i16)
  n167 = To Word Integer(number=w53) -> (16bit integer=w56:i16)
  n168 = To Word Integer(number=w54) -> (16bit integer=w57:i16)
  n169 = Add(x=w47, y=w50) -> (x+y=w49:i16)
  n170 = Compound Arithmetic op=ADD(w58, w56, w57, i16 12 ("y")) -> (w52:i16)
  n171 = Bundle By Name(cluster=w45, "Right"=w49, "Bottom"=w52) -> (w46:T13)
  n172 = property class="VI"(reference=w44, "Front Panel.PanelBounds"=w46) -> ()  [unwired: 1 in, 2 out]
